vi "grab image_2_sow2.vi"(8 "ErrorIn":errorcluster, 9 "Image number":u32, 10 "BuffNr":i16, 11 "ph":u64) -> (0 "output image":u16[][](array[numeric]), 1 "error out":errorcluster, 2 "Buffer_Ready":bool, 3 "hout":u64)   [LabVIEW 2014]
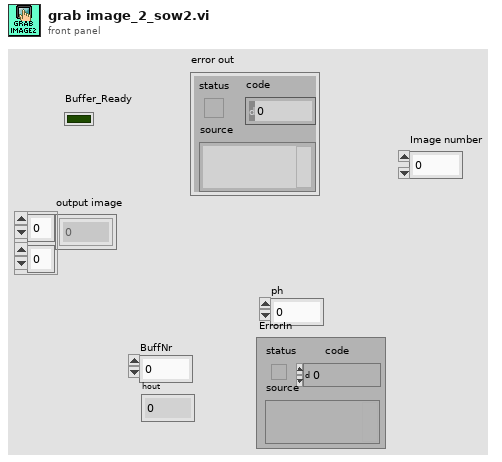
[diagram p1: front panel]
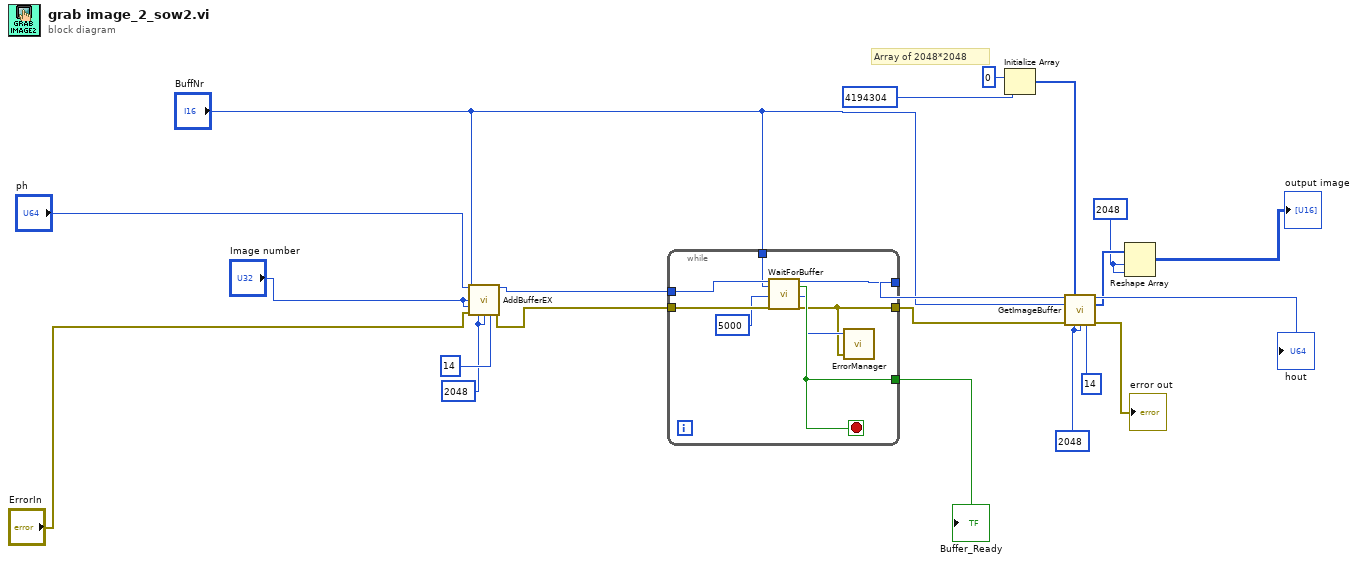
[diagram p0: block diagram]
diagram:
  w2 = u16 2048 ("xRes")
  w10 = 2048
  w14 = u16 2048
  # "Array of 2048*2048"
  n1 = call <userlib>:"AddBufferEX.vi"("ph"="ph", "BuffNr"="BuffNr", "1stImage"="Image number", "LastImage"="Image number", "error in (no error)"="ErrorIn", "XRes"=w14, "YRes"=w14, "BitPerPixel"=u16 14) -> ("hout"=w9:u64, "error out"=w8:errorcluster)  [unwired: 5 in, 1 out]
  n2 = while {
    tunnel: w9 -> [w29]
    tunnel: w8 -> [w28]
    tunnel: [w26] -> w13
    tunnel: [w22] -> w12
    tunnel: "BuffNr" -> [w25]
    tunnel: [w24] -> w5
    stop <- w24 stop-if-true
    n3 = call <userlib>:"WaitForBuffer.vi"("ph"=w29, "sBufNr"=w25, "timeout"=u32 5000, "error in (no error)"=w28) -> ("hout"=w26:u64, "Buffer_Ready"=w24:bool, "ErrorCode"=w23:i32, "error out"=w22:errorcluster)  [unwired: 11 in, 1 out]
    n4 = call <userlib>:"ErrorManager.vi"("ErrorIn"=w22, "ErrorCode"=w23) -> ()  [unwired: 3 in, 1 out]
  }
  "Buffer_Ready" <- w5
  n5 = Initialize Array(i16 0 ("element"), 4194304 ("dimension size")) -> (w18:i16[])
  n6 = call <userlib>:"GetImageBuffer.vi"("ph"=w13, "BuffIn"=w18, "BuffNr"="BuffNr", "error in (no error)"=w12, "xRes"=w2, "yRes"=w2, "Bitresolution"=u16 14 ("BitPerPixel")) -> ("hout"=→"hout":u64, "BuffOut"=w11:u16[], "error out"=→"error out":errorcluster)  [unwired: 5 in, 1 out]
  n7 = Reshape Array(w11, w10, w10) -> (→"output image":u16[][])
